vi "NIMS_NS_iir_lpnorm.vi"(5 "Function name":string, 6 "Line number":i32, 7 "Number of outputs requested":i32, 8 "error in (no error)":errorcluster, 11 "[A]":variant[](array[variant])) -> (0 "error out":errorcluster, 3 "[funct(A)]":variant[](array[variant]))   [LabVIEW 2017]
uses:
  <vilib>/imath/engines/lvmath/Functions/Error Handling/error.ctl
  <instcachedir>/0/NIMS_RunTimeType_From StrictType (excl LVString)_1019F277F0A747EDBCA0F6C52CA54500.lvgen/NIMS_RunTimeType_From StrictType (excl LVString)_1019F277F0A747EDBCA0F6C52CA54500_000.vi
  <instcachedir>/0/NIMS_Get Scalar_w Error_1987D997E87247DDAC16EA23A5E9E4FC.lvgen/NIMS_Get Scalar_w Error_1987D997E87247DDAC16EA23A5E9E4FC_000.vi
  <instcachedir>/0/NIMS_Complex To Real_BE01396FDE034E8E94CEBBA1E368668D.lvgen/NIMS_Complex To Real_BE01396FDE034E8E94CEBBA1E368668D_000.vi
  <instcachedir>/0/NIMS_Get Any Vector_w Error - Matrix_9FDB8FBE264C42EDBC8FF9BA66C3EF33.lvgen/NIMS_Get Any Vector_w Error - Matrix_9FDB8FBE264C42EDBC8FF9BA66C3EF33_001.vi
  <instcachedir>/0/NIMS_RunTimeType_To Numeric_1CBDAFC4EFAD4045A1DE52278D16738D.lvgen/NIMS_RunTimeType_To Numeric_1CBDAFC4EFAD4045A1DE52278D16738D_000.vi
  <vilib>/addons/Digital Filter Design/NI_DigFilter_MathScript.lvlib
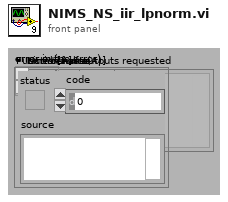
[diagram p1: front panel]
types:
  T1 = typedef "error.ctl" = enum16{"No Error", "Problem", "Input type must not be void", "Incorrect number of parameters", "Function not defined for non-numeric types", "An output variable of the user-defined function is undefined", "Function only defined for character arrays", "Function not defined for boolean, character, or single precision", "Function not defined for complex types", "Not a valid operation", "Inputs must be scalar", "Input matrices are not the same size", "Function only available on RT", "Input matrices must be nonnegative integers of the same type", "Arguments must be non-negative integers less than bitmax", "Number to complement must be less than 2^N", "Bit to get is outside range", "Bit to set is outside range", "Input must be real type ", "At least one parameter must be scalar", "Unable to display plug-in data on RT", "Function not defined for higher dimensional matrices", "Invalid attributes", "Wrong Type of Input Arguments", "Wrong Argument Option", "Invalid file identifier", "Indices must be real positive integers", "The variable is not a matrix data type.", "Number of elements must be the same for indices and values", "You cannot replace elements of a matrix with non-matrix data types.", "Cannot resize a 2D matrix with a linear index", "Unknown variable or symbol", "Indices out of range", "Empty matrix deletion can not be used with two indices", "Number of rows and columns must be the same for indices and values.", "Complex cannot be converted to Boolean", "Char cannot be converted to Boolean", "int64 cannot be converted to Boolean", "uint64 cannot be converted to Boolean", "You cannot convert a Boolean to a character.", "Incompatible input size in 3D surface function", "All rows must have the same number of columns", "Incompatible types", "Invalid matrix dimensions", "Dimension must be 1 or 2", "Base must be an integer between 2 and 36", "Invalid input", "Square matrix required", "Function 'timerstart' must be called before 'timerstop'", "Arguments must be positive real", "Step must not be zero", "Wrong number of input arguments", "Wrong number of output arguments", "Too many index arguments", "Input scalar must be >= 0", "Input scalar must be positive", "Input scalar must not be 0", "Input scalar must be in range [0,1]", "Can't use conditionally defined variable that's undefined", "Input must be a vector", "RT Exec Trace Toolkit not licensed", "Empty vector error", "All elements must be in domain [-1,1]", "All real elements of input vector must be >= 0", "All elements of input vector must be positive", "Values of input vectors are not compatible", "DAQmx not installed", "Input vector must be an increasing vector", "Dereferenced field does not exist within the struct", "A vector or matrix of structures must be indexed before it can be dereferenced", "Lenths of two input vectors are not compatible", "Invalid fieldname", "Empty matrix error", "Cannot use '.' on a type other than Struct", "Unused074", "Data type of the struct's field name is invalid", "Using . to dereference data that is not a struct", "Input struct contains invalid type ", "Size of input matrix is incompatible with input size", "Invalid format specifier", "Could not find field within struct", "Bad permutation array", "Mismatched fieldnames", "ode: User Function could not be opened", "ode: User Function signature does not meet ode requirements", "Unused085", "RunTime: MathScript could not be compiled", "Unknown function", "Only scalars and strings supported", "ode: User Function signature has incorrect number of inputs", "ode:User Function signature has incorrect number of outputs", "Range is too large", "End used without variable", "Function not available (RTE)", "Custom user error", "Arguments must be integers less than bitmax", "Shared library not found", "Header file not found", "Shared library already loaded", "Shared library not loaded", "Shared library function not found", "Shared library string return problem", "Problem calling shared library function", "Problem loading shared library from OS", "Problem parsing shared library header file", "Shared library incompatible types", "Shared library unsupported return type", "Shared library function not exported", "Shared library unsupported input type", "Problem unloading shared library from OS", "Function only available from UI", "Function specified in argument is missing", "An internal error has occurred", "Invalid object", "Invalid property", "Read-only property", "A break command has occurred", "A continue command has occurred", "A return command has occurred", "ode: times parameter invalid", "Function specified in argument has incorrect signature", "Function not found in file", "Reserved keyword cannot be defined as variable", "Reserved keyword cannot be defined as a function or script", "Arguments must be string literals", "Function not supported on this platform", "All columns must have the same number of rows", "Function ignored in RTE warning", "Cannot use : as a parameter that is not a variable", "Output can't be coerced to requested type", "Function not supported on current target", "Variable dependent on an unwired function input", "Unused132", "Unused133", "Unused134", "Unused135", "Unused136", "Unused137", "Unused138", "Unused139", "Global/Persistent must only take constants as arguments.", "Varargin must be last input in the function definition.", "Varargout must be last output in the function definition.", "Invalid output type. Cannot output a cell array of any type other than string.", "Invalid output type. Type is a dynamic struct.", "Invalid output type. Type is a struct that has a field whose type is not known until run-time", "Invalid output type. Type is a struct that has a field which is a plot object.", "MathScript parser DLL missing", "MathScript requires LabVIEW Full", "MathScript license is invalid or missing", "Varargout not supported except in assignments."}
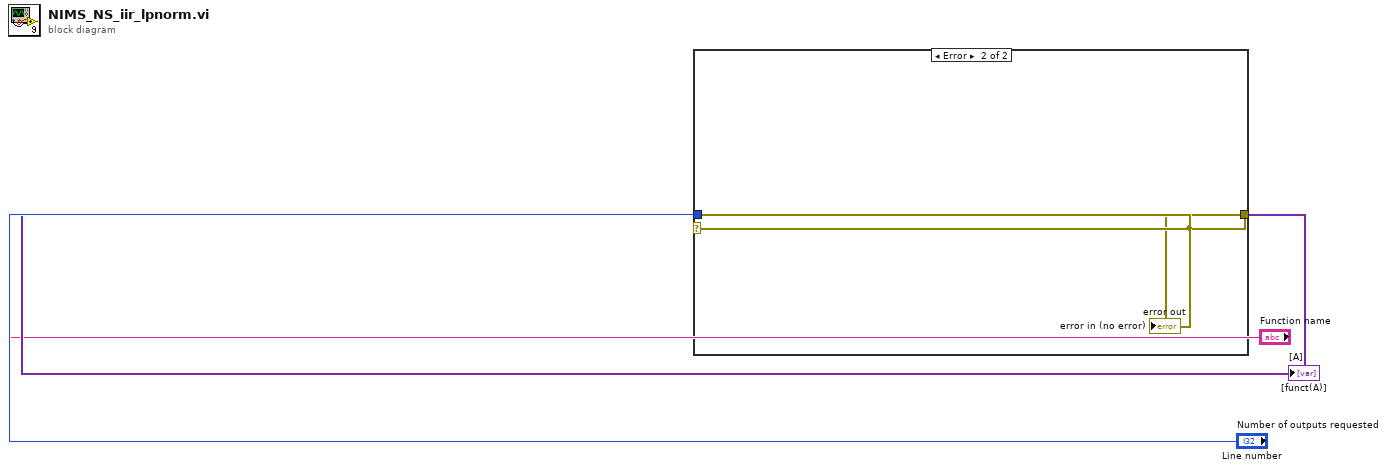
[diagram p0: block diagram]
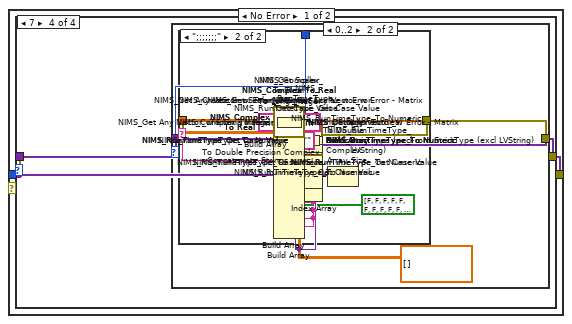
[diagram p2: hidden frame]
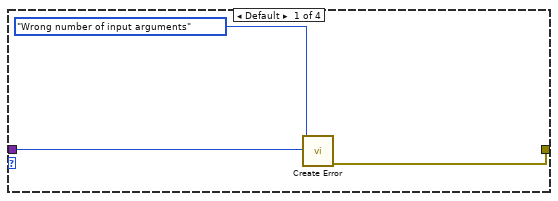
[diagram p3: hidden frame]
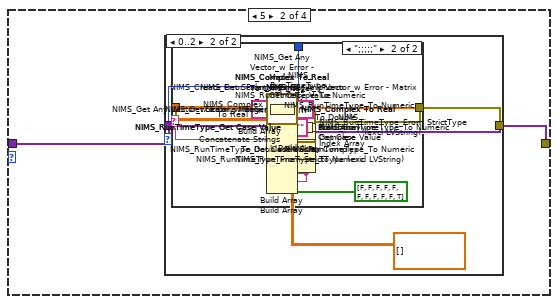
[diagram p4: hidden frame]
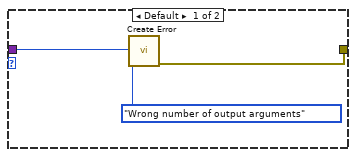
[diagram p5: hidden frame]
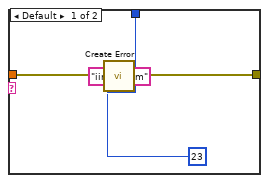
[diagram p6: hidden frame]
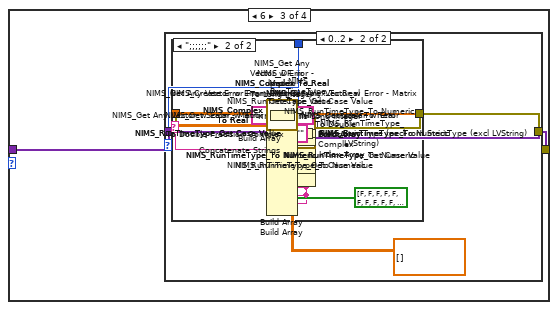
[diagram p7: hidden frame]
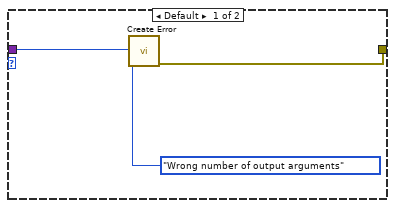
[diagram p8: hidden frame]
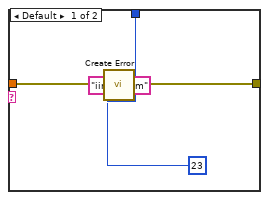
[diagram p9: hidden frame]
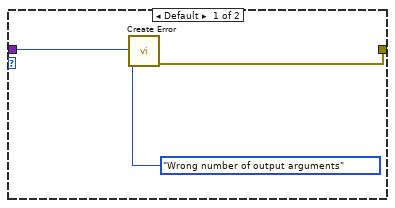
[diagram p10: hidden frame]
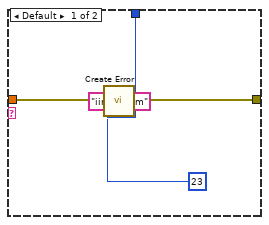
[diagram p11: hidden frame]
diagram:
  n1 = case shown="Error" "error in (no error)" {
    selector: "error in (no error)" -> [_ w322]
    tunnel: [w15 _] -> w4
    tunnel: [w14 w322] -> w3
    tunnel: "error in (no error)" -> [w13 _]
    tunnel: "Number of outputs requested" -> [w12 _]
    tunnel: "[A]" -> [w11 _]
    tunnel: "Function name" -> [w10 _]
    tunnel: "Line number" -> [w9 _]
    frame No Error {
      n2 = Array Size(array=w11) -> (size(s)=w8:i32)
      n3 = case shown="7" w8 {
        tunnel: [_ w27 w118 w218] -> w15
        tunnel: w10 -> [w19 w24 w115 w215]
        tunnel: w9 -> [w20 w25 w116 w216]
        tunnel: w13 -> [w17 w23 w114 w214]
        tunnel: [w16 w22 w113 w213] -> w14
        tunnel: w12 -> [_ w21 w112 w212]
        tunnel: w11 -> [_ w26 w117 w217]
        frame Default {
          n4 = call <vilib>:"Create Error.vi"("Function name"=w19, "error in (no error)"=w17, "Error Enum"=error."Wrong number of input arguments", "Line number"=w20) -> ("error out"=w16:errorcluster)  [unwired: 6 in, 1 out]
        }
        frame 5 {
          n5 = case shown="0..2" w21 {
            tunnel: [_ w33] -> w27
            tunnel: w24 -> [w31 _]
            tunnel: w25 -> [w32 w67]
            tunnel: w23 -> [w29 w65]
            tunnel: [w28 w44] -> w22
            tunnel: w26 -> [_ w68]
            frame Default {
              n6 = call <vilib>:"Create Error.vi"("Function name"=w31, "error in (no error)"=w29, "Error Enum"=error."Wrong number of output arguments", "Line number"=w32) -> ("error out"=w28:errorcluster)  [unwired: 6 in, 1 out]
            }
            frame 0..2 {
              n7 = Index Array(array=w68) -> (element #1=w64:variant, element #2=w60:variant, element #3=w56:variant, element #4=w52:variant, element #5=w48:variant)  [unwired: 5 in]
              n8 = call <vilib>:"NIMS_RunTimeType_Get Case Value.vi"("Data In"=w48) -> ("Case Value"=w45:string)  [unwired: 9 in, 1 out]
              n9 = call-generic <vilib>:"NIMS_RunTimeType_To Numeric.vi"("DataType"=cdb[][] [], "Variant"=w48) -> ("data"=w46:cdb[][])  [unwired: 1 in]
              n10 = call <vilib>:"NIMS_RunTimeType_Get Case Value.vi"("Data In"=w52) -> ("Case Value"=w49:string)  [unwired: 9 in, 1 out]
              n11 = call-generic <vilib>:"NIMS_RunTimeType_To Numeric.vi"("DataType"=cdb[][] [], "Variant"=w52) -> ("data"=w50:cdb[][])  [unwired: 1 in]
              n12 = call <vilib>:"NIMS_RunTimeType_Get Case Value.vi"("Data In"=w56) -> ("Case Value"=w53:string)  [unwired: 9 in, 1 out]
              n13 = call-generic <vilib>:"NIMS_RunTimeType_To Numeric.vi"("DataType"=cdb[][] [], "Variant"=w56) -> ("data"=w54:cdb[][])  [unwired: 1 in]
              n14 = call <vilib>:"NIMS_RunTimeType_Get Case Value.vi"("Data In"=w60) -> ("Case Value"=w57:string)  [unwired: 9 in, 1 out]
              n15 = call-generic <vilib>:"NIMS_RunTimeType_To Numeric.vi"("DataType"=cdb[][] [], "Variant"=w60) -> ("data"=w58:cdb[][])  [unwired: 1 in]
              n16 = call <vilib>:"NIMS_RunTimeType_Get Case Value.vi"("Data In"=w64) -> ("Case Value"=w61:string)  [unwired: 9 in, 1 out]
              n17 = call-generic <vilib>:"NIMS_RunTimeType_To Numeric.vi"("DataType"=cdb[][] [], "Variant"=w64) -> ("data"=w62:cdb[][])  [unwired: 1 in]
              n18 = Concatenate Strings(w61, w57, w53, w49, w45) -> (w66:string)
              n19 = case shown="\";;;;;\"" w66 {
                tunnel: w65 -> [w70 w80]
                tunnel: [_ w75] -> w43
                tunnel: [_ w74] -> w39
                tunnel: [w69 w76] -> w44
                tunnel: w62 -> [_ w110]
                tunnel: w58 -> [_ w106]
                tunnel: w54 -> [_ w102]
                tunnel: w50 -> [_ w99]
                tunnel: w46 -> [_ w96]
                tunnel: w67 -> [w73 w83]
                frame Default {
                  n20 = call <vilib>:"Create Error.vi"("Function name"="iir_lpnorm", "error in (no error)"=w70, "Error Enum"=23, "Line number"=w73) -> ("error out"=w69:errorcluster)  [unwired: 6 in, 1 out]
                }
                frame ";;;;;" {
                  w78 = "iir_lpnorm"
                  n21 = call-generic <vilib>:"NIMS_Complex To Real.vi"("A"=w96) -> ("Error Enum"=w86:T1, "Real(A)"=w95:dbl[][])  [unwired: 8 in, 1 out]
                  n22 = call-generic <vilib>:"NIMS_Get Any Vector_w Error - Matrix.vi"("A"=w95) -> ("Error Enum"=w85:T1, "Vector"=w97:dbl[])  [unwired: 8 in, 1 out]
                  n23 = call-generic <vilib>:"NIMS_Complex To Real.vi"("A"=w99) -> ("Error Enum"=w88:T1, "Real(A)"=w98:dbl[][])  [unwired: 8 in, 1 out]
                  n24 = call-generic <vilib>:"NIMS_Get Any Vector_w Error - Matrix.vi"("A"=w98) -> ("Error Enum"=w87:T1, "Vector"=w100:dbl[])  [unwired: 8 in, 1 out]
                  n25 = call-generic <vilib>:"NIMS_Complex To Real.vi"("A"=w102) -> ("Error Enum"=w90:T1, "Real(A)"=w101:dbl[][])  [unwired: 8 in, 1 out]
                  n26 = call-generic <vilib>:"NIMS_Get Any Vector_w Error - Matrix.vi"("A"=w101) -> ("Error Enum"=w89:T1, "Vector"=w103:dbl[])  [unwired: 8 in, 1 out]
                  n27 = call-generic <vilib>:"NIMS_Complex To Real.vi"("A"=w106) -> ("Error Enum"=w92:T1, "Real(A)"=w105:dbl[][])  [unwired: 8 in, 1 out]
                  n28 = To Long Integer(number=w105) -> (32bit integer=w104:i32[][])
                  n29 = call-generic <vilib>:"NIMS_Get Scalar_w Error.vi"("A"=w104) -> ("Error Enum"=w91:T1, "Scalar"=w107:i32)  [unwired: 8 in, 1 out]
                  n30 = call-generic <vilib>:"NIMS_Complex To Real.vi"("A"=w110) -> ("Error Enum"=w94:T1, "Real(A)"=w109:dbl[][])  [unwired: 8 in, 1 out]
                  n31 = To Long Integer(number=w109) -> (32bit integer=w108:i32[][])
                  n32 = call-generic <vilib>:"NIMS_Get Scalar_w Error.vi"("A"=w108) -> ("Error Enum"=w93:T1, "Scalar"=w111:i32)  [unwired: 8 in, 1 out]
                  n33 = call <vilib>:"NIMS_DF_iir_lpnorm.vi"("mag"=w97, "e"=w100, "f"=w103, "d"=w107, "n"=w111) -> ("error"=w84:i32, "a"=w74:dbl[], "b"=w75:dbl[])  [unwired: 4 in]
                  n34 = Build Array(w78, w78, w78, w78, w78, w78, w78, w78, w78, w78, "iir_lpnorm") -> (w81:string[])
                  n35 = Build Array(w94, w93, w92, w91, w90, w89, w88, w87, w86, w85, w84) -> (w82:i32[])
                  n36 = call <vilib>:"NIMS_Create Error From Enums.vi"("Error Code"=bool[] [FALSE, FALSE, FALSE, FALSE, FALSE, FALSE, FALSE, FALSE, FALSE, FALSE, TRUE], "error in (no error)"=w80, "Line no"=w83, "Error Enums"=w82, "Function names"=w81) -> ("error out"=w76:errorcluster)  [unwired: 6 in]
                }
              }
              n37 = Build Array(w39) -> (w38:dbl[][])
              n38 = To Double Precision Complex(1:w38) -> (0:w37:cdb[][])
              n39 = call-generic <vilib>:"NIMS_RunTimeType_From StrictType (excl LVString).vi"("Plug-In Name"="", "Data In"=w37) -> ("Data Out"=w34:variant)  [unwired: 2 in]
              n40 = Build Array(w43) -> (w42:dbl[][])
              n41 = To Double Precision Complex(1:w42) -> (0:w41:cdb[][])
              n42 = call-generic <vilib>:"NIMS_RunTimeType_From StrictType (excl LVString).vi"("Plug-In Name"="", "Data In"=w41) -> ("Data Out"=w35:variant)  [unwired: 2 in]
              n43 = Build Array(w35, w34) -> (w33:variant[])
            }
          }
        }
        frame 6 {
          n44 = case shown="0..2" w112 {
            tunnel: [_ w124] -> w118
            tunnel: w115 -> [w122 _]
            tunnel: w116 -> [w123 w162]
            tunnel: w114 -> [w120 w160]
            tunnel: [w119 w135] -> w113
            tunnel: w117 -> [_ w163]
            frame Default {
              n45 = call <vilib>:"Create Error.vi"("Function name"=w122, "error in (no error)"=w120, "Error Enum"=error."Wrong number of output arguments", "Line number"=w123) -> ("error out"=w119:errorcluster)  [unwired: 6 in, 1 out]
            }
            frame 0..2 {
              n46 = Index Array(array=w163) -> (element #1=w159:variant, element #2=w155:variant, element #3=w151:variant, element #4=w147:variant, element #5=w143:variant, element #6=w139:variant)  [unwired: 6 in]
              n47 = call <vilib>:"NIMS_RunTimeType_Get Case Value.vi"("Data In"=w139) -> ("Case Value"=w136:string)  [unwired: 9 in, 1 out]
              n48 = call-generic <vilib>:"NIMS_RunTimeType_To Numeric.vi"("DataType"=cdb[][] [], "Variant"=w139) -> ("data"=w137:cdb[][])  [unwired: 1 in]
              n49 = call <vilib>:"NIMS_RunTimeType_Get Case Value.vi"("Data In"=w143) -> ("Case Value"=w140:string)  [unwired: 9 in, 1 out]
              n50 = call-generic <vilib>:"NIMS_RunTimeType_To Numeric.vi"("DataType"=cdb[][] [], "Variant"=w143) -> ("data"=w141:cdb[][])  [unwired: 1 in]
              n51 = call <vilib>:"NIMS_RunTimeType_Get Case Value.vi"("Data In"=w147) -> ("Case Value"=w144:string)  [unwired: 9 in, 1 out]
              n52 = call-generic <vilib>:"NIMS_RunTimeType_To Numeric.vi"("DataType"=cdb[][] [], "Variant"=w147) -> ("data"=w145:cdb[][])  [unwired: 1 in]
              n53 = call <vilib>:"NIMS_RunTimeType_Get Case Value.vi"("Data In"=w151) -> ("Case Value"=w148:string)  [unwired: 9 in, 1 out]
              n54 = call-generic <vilib>:"NIMS_RunTimeType_To Numeric.vi"("DataType"=cdb[][] [], "Variant"=w151) -> ("data"=w149:cdb[][])  [unwired: 1 in]
              n55 = call <vilib>:"NIMS_RunTimeType_Get Case Value.vi"("Data In"=w155) -> ("Case Value"=w152:string)  [unwired: 9 in, 1 out]
              n56 = call-generic <vilib>:"NIMS_RunTimeType_To Numeric.vi"("DataType"=cdb[][] [], "Variant"=w155) -> ("data"=w153:cdb[][])  [unwired: 1 in]
              n57 = call <vilib>:"NIMS_RunTimeType_Get Case Value.vi"("Data In"=w159) -> ("Case Value"=w156:string)  [unwired: 9 in, 1 out]
              n58 = call-generic <vilib>:"NIMS_RunTimeType_To Numeric.vi"("DataType"=cdb[][] [], "Variant"=w159) -> ("data"=w157:cdb[][])  [unwired: 1 in]
              n59 = Concatenate Strings(w156, w152, w148, w144, w140, w136) -> (w161:string)
              n60 = case shown="\";;;;;;\"" w161 {
                tunnel: w160 -> [w165 w175]
                tunnel: [_ w170] -> w134
                tunnel: [_ w169] -> w130
                tunnel: [w164 w171] -> w135
                tunnel: w157 -> [_ w210]
                tunnel: w153 -> [_ w206]
                tunnel: w149 -> [_ w202]
                tunnel: w145 -> [_ w199]
                tunnel: w141 -> [_ w196]
                tunnel: w137 -> [_ w193]
                tunnel: w162 -> [w168 w178]
                frame Default {
                  n61 = call <vilib>:"Create Error.vi"("Function name"="iir_lpnorm", "error in (no error)"=w165, "Error Enum"=23, "Line number"=w168) -> ("error out"=w164:errorcluster)  [unwired: 6 in, 1 out]
                }
                frame ";;;;;;" {
                  w173 = "iir_lpnorm"
                  n62 = call-generic <vilib>:"NIMS_Complex To Real.vi"("A"=w193) -> ("Error Enum"=w181:T1, "Real(A)"=w192:dbl[][])  [unwired: 8 in, 1 out]
                  n63 = call-generic <vilib>:"NIMS_Get Any Vector_w Error - Matrix.vi"("A"=w192) -> ("Error Enum"=w180:T1, "Vector"=w194:dbl[])  [unwired: 8 in, 1 out]
                  n64 = call-generic <vilib>:"NIMS_Complex To Real.vi"("A"=w196) -> ("Error Enum"=w183:T1, "Real(A)"=w195:dbl[][])  [unwired: 8 in, 1 out]
                  n65 = call-generic <vilib>:"NIMS_Get Any Vector_w Error - Matrix.vi"("A"=w195) -> ("Error Enum"=w182:T1, "Vector"=w197:dbl[])  [unwired: 8 in, 1 out]
                  n66 = call-generic <vilib>:"NIMS_Complex To Real.vi"("A"=w199) -> ("Error Enum"=w185:T1, "Real(A)"=w198:dbl[][])  [unwired: 8 in, 1 out]
                  n67 = call-generic <vilib>:"NIMS_Get Any Vector_w Error - Matrix.vi"("A"=w198) -> ("Error Enum"=w184:T1, "Vector"=w200:dbl[])  [unwired: 8 in, 1 out]
                  n68 = call-generic <vilib>:"NIMS_Complex To Real.vi"("A"=w202) -> ("Error Enum"=w187:T1, "Real(A)"=w201:dbl[][])  [unwired: 8 in, 1 out]
                  n69 = call-generic <vilib>:"NIMS_Get Any Vector_w Error - Matrix.vi"("A"=w201) -> ("Error Enum"=w186:T1, "Vector"=w203:dbl[])  [unwired: 8 in, 1 out]
                  n70 = call-generic <vilib>:"NIMS_Complex To Real.vi"("A"=w206) -> ("Error Enum"=w189:T1, "Real(A)"=w205:dbl[][])  [unwired: 8 in, 1 out]
                  n71 = To Long Integer(number=w205) -> (32bit integer=w204:i32[][])
                  n72 = call-generic <vilib>:"NIMS_Get Scalar_w Error.vi"("A"=w204) -> ("Error Enum"=w188:T1, "Scalar"=w207:i32)  [unwired: 8 in, 1 out]
                  n73 = call-generic <vilib>:"NIMS_Complex To Real.vi"("A"=w210) -> ("Error Enum"=w191:T1, "Real(A)"=w209:dbl[][])  [unwired: 8 in, 1 out]
                  n74 = To Long Integer(number=w209) -> (32bit integer=w208:i32[][])
                  n75 = call-generic <vilib>:"NIMS_Get Scalar_w Error.vi"("A"=w208) -> ("Error Enum"=w190:T1, "Scalar"=w211:i32)  [unwired: 8 in, 1 out]
                  n76 = call <vilib>:"NIMS_DF_iir_lpnorm.vi"("w"=w194, "mag"=w197, "e"=w200, "f"=w203, "d"=w207, "n"=w211) -> ("error"=w179:i32, "a"=w169:dbl[], "b"=w170:dbl[])  [unwired: 3 in]
                  n77 = Build Array(w173, w173, w173, w173, w173, w173, w173, w173, w173, w173, w173, w173, "iir_lpnorm") -> (w176:string[])
                  n78 = Build Array(w191, w190, w189, w188, w187, w186, w185, w184, w183, w182, w181, w180, w179) -> (w177:i32[])
                  n79 = call <vilib>:"NIMS_Create Error From Enums.vi"("Error Code"=bool[] [FALSE, FALSE, FALSE, FALSE, FALSE, FALSE, FALSE, FALSE, FALSE, FALSE, FALSE, FALSE, TRUE], "error in (no error)"=w175, "Line no"=w178, "Error Enums"=w177, "Function names"=w176) -> ("error out"=w171:errorcluster)  [unwired: 6 in]
                }
              }
              n80 = Build Array(w130) -> (w129:dbl[][])
              n81 = To Double Precision Complex(1:w129) -> (0:w128:cdb[][])
              n82 = call-generic <vilib>:"NIMS_RunTimeType_From StrictType (excl LVString).vi"("Plug-In Name"="", "Data In"=w128) -> ("Data Out"=w125:variant)  [unwired: 2 in]
              n83 = Build Array(w134) -> (w133:dbl[][])
              n84 = To Double Precision Complex(1:w133) -> (0:w132:cdb[][])
              n85 = call-generic <vilib>:"NIMS_RunTimeType_From StrictType (excl LVString).vi"("Plug-In Name"="", "Data In"=w132) -> ("Data Out"=w126:variant)  [unwired: 2 in]
              n86 = Build Array(w126, w125) -> (w124:variant[])
            }
          }
        }
        frame 7 {
          n87 = case shown="0..2" w212 {
            tunnel: [_ w224] -> w218
            tunnel: w215 -> [w222 _]
            tunnel: w216 -> [w223 w266]
            tunnel: w214 -> [w220 w264]
            tunnel: [w219 w235] -> w213
            tunnel: w217 -> [_ w267]
            frame Default {
              n88 = call <vilib>:"Create Error.vi"("Function name"=w222, "error in (no error)"=w220, "Error Enum"=error."Wrong number of output arguments", "Line number"=w223) -> ("error out"=w219:errorcluster)  [unwired: 6 in, 1 out]
            }
            frame 0..2 {
              n89 = Index Array(array=w267) -> (element #1=w263:variant, element #2=w259:variant, element #3=w255:variant, element #4=w251:variant, element #5=w247:variant, element #6=w243:variant, element #7=w239:variant)  [unwired: 7 in]
              n90 = call <vilib>:"NIMS_RunTimeType_Get Case Value.vi"("Data In"=w239) -> ("Case Value"=w236:string)  [unwired: 9 in, 1 out]
              n91 = call-generic <vilib>:"NIMS_RunTimeType_To Numeric.vi"("DataType"=cdb[][] [], "Variant"=w239) -> ("data"=w237:cdb[][])  [unwired: 1 in]
              n92 = call <vilib>:"NIMS_RunTimeType_Get Case Value.vi"("Data In"=w243) -> ("Case Value"=w240:string)  [unwired: 9 in, 1 out]
              n93 = call-generic <vilib>:"NIMS_RunTimeType_To Numeric.vi"("DataType"=cdb[][] [], "Variant"=w243) -> ("data"=w241:cdb[][])  [unwired: 1 in]
              n94 = call <vilib>:"NIMS_RunTimeType_Get Case Value.vi"("Data In"=w247) -> ("Case Value"=w244:string)  [unwired: 9 in, 1 out]
              n95 = call-generic <vilib>:"NIMS_RunTimeType_To Numeric.vi"("DataType"=cdb[][] [], "Variant"=w247) -> ("data"=w245:cdb[][])  [unwired: 1 in]
              n96 = call <vilib>:"NIMS_RunTimeType_Get Case Value.vi"("Data In"=w251) -> ("Case Value"=w248:string)  [unwired: 9 in, 1 out]
              n97 = call-generic <vilib>:"NIMS_RunTimeType_To Numeric.vi"("DataType"=cdb[][] [], "Variant"=w251) -> ("data"=w249:cdb[][])  [unwired: 1 in]
              n98 = call <vilib>:"NIMS_RunTimeType_Get Case Value.vi"("Data In"=w255) -> ("Case Value"=w252:string)  [unwired: 9 in, 1 out]
              n99 = call-generic <vilib>:"NIMS_RunTimeType_To Numeric.vi"("DataType"=cdb[][] [], "Variant"=w255) -> ("data"=w253:cdb[][])  [unwired: 1 in]
              n100 = call <vilib>:"NIMS_RunTimeType_Get Case Value.vi"("Data In"=w259) -> ("Case Value"=w256:string)  [unwired: 9 in, 1 out]
              n101 = call-generic <vilib>:"NIMS_RunTimeType_To Numeric.vi"("DataType"=cdb[][] [], "Variant"=w259) -> ("data"=w257:cdb[][])  [unwired: 1 in]
              n102 = call <vilib>:"NIMS_RunTimeType_Get Case Value.vi"("Data In"=w263) -> ("Case Value"=w260:string)  [unwired: 9 in, 1 out]
              n103 = call-generic <vilib>:"NIMS_RunTimeType_To Numeric.vi"("DataType"=cdb[][] [], "Variant"=w263) -> ("data"=w261:cdb[][])  [unwired: 1 in]
              n104 = Concatenate Strings(w260, w256, w252, w248, w244, w240, w236) -> (w265:string)
              n105 = case shown="\";;;;;;;\"" w265 {
                tunnel: w264 -> [w269 w279]
                tunnel: [_ w274] -> w234
                tunnel: [_ w273] -> w230
                tunnel: [w268 w275] -> w235
                tunnel: w261 -> [_ w320]
                tunnel: w257 -> [_ w316]
                tunnel: w253 -> [_ w312]
                tunnel: w249 -> [_ w309]
                tunnel: w245 -> [_ w306]
                tunnel: w241 -> [_ w303]
                tunnel: w237 -> [_ w300]
                tunnel: w266 -> [w272 w282]
                frame Default {
                  n106 = call <vilib>:"Create Error.vi"("Function name"="iir_lpnorm", "error in (no error)"=w269, "Error Enum"=23, "Line number"=w272) -> ("error out"=w268:errorcluster)  [unwired: 6 in, 1 out]
                }
                frame ";;;;;;;" {
                  w277 = "iir_lpnorm"
                  n107 = call-generic <vilib>:"NIMS_Complex To Real.vi"("A"=w300) -> ("Error Enum"=w285:T1, "Real(A)"=w299:dbl[][])  [unwired: 8 in, 1 out]
                  n108 = To Long Integer(number=w299) -> (32bit integer=w298:i32[][])
                  n109 = call-generic <vilib>:"NIMS_Get Scalar_w Error.vi"("A"=w298) -> ("Error Enum"=w284:T1, "Scalar"=w301:i32)  [unwired: 8 in, 1 out]
                  n110 = call-generic <vilib>:"NIMS_Complex To Real.vi"("A"=w303) -> ("Error Enum"=w287:T1, "Real(A)"=w302:dbl[][])  [unwired: 8 in, 1 out]
                  n111 = call-generic <vilib>:"NIMS_Get Any Vector_w Error - Matrix.vi"("A"=w302) -> ("Error Enum"=w286:T1, "Vector"=w304:dbl[])  [unwired: 8 in, 1 out]
                  n112 = call-generic <vilib>:"NIMS_Complex To Real.vi"("A"=w306) -> ("Error Enum"=w289:T1, "Real(A)"=w305:dbl[][])  [unwired: 8 in, 1 out]
                  n113 = call-generic <vilib>:"NIMS_Get Any Vector_w Error - Matrix.vi"("A"=w305) -> ("Error Enum"=w288:T1, "Vector"=w307:dbl[])  [unwired: 8 in, 1 out]
                  n114 = call-generic <vilib>:"NIMS_Complex To Real.vi"("A"=w309) -> ("Error Enum"=w291:T1, "Real(A)"=w308:dbl[][])  [unwired: 8 in, 1 out]
                  n115 = call-generic <vilib>:"NIMS_Get Any Vector_w Error - Matrix.vi"("A"=w308) -> ("Error Enum"=w290:T1, "Vector"=w310:dbl[])  [unwired: 8 in, 1 out]
                  n116 = call-generic <vilib>:"NIMS_Complex To Real.vi"("A"=w312) -> ("Error Enum"=w293:T1, "Real(A)"=w311:dbl[][])  [unwired: 8 in, 1 out]
                  n117 = call-generic <vilib>:"NIMS_Get Any Vector_w Error - Matrix.vi"("A"=w311) -> ("Error Enum"=w292:T1, "Vector"=w313:dbl[])  [unwired: 8 in, 1 out]
                  n118 = call-generic <vilib>:"NIMS_Complex To Real.vi"("A"=w316) -> ("Error Enum"=w295:T1, "Real(A)"=w315:dbl[][])  [unwired: 8 in, 1 out]
                  n119 = To Long Integer(number=w315) -> (32bit integer=w314:i32[][])
                  n120 = call-generic <vilib>:"NIMS_Get Scalar_w Error.vi"("A"=w314) -> ("Error Enum"=w294:T1, "Scalar"=w317:i32)  [unwired: 8 in, 1 out]
                  n121 = call-generic <vilib>:"NIMS_Complex To Real.vi"("A"=w320) -> ("Error Enum"=w297:T1, "Real(A)"=w319:dbl[][])  [unwired: 8 in, 1 out]
                  n122 = To Long Integer(number=w319) -> (32bit integer=w318:i32[][])
                  n123 = call-generic <vilib>:"NIMS_Get Scalar_w Error.vi"("A"=w318) -> ("Error Enum"=w296:T1, "Scalar"=w321:i32)  [unwired: 8 in, 1 out]
                  n124 = call <vilib>:"NIMS_DF_iir_lpnorm.vi"("p"=w301, "w"=w304, "mag"=w307, "e"=w310, "f"=w313, "d"=w317, "n"=w321) -> ("error"=w283:i32, "a"=w273:dbl[], "b"=w274:dbl[])  [unwired: 2 in]
                  n125 = Build Array(w277, w277, w277, w277, w277, w277, w277, w277, w277, w277, w277, w277, w277, w277, "iir_lpnorm") -> (w280:string[])
                  n126 = Build Array(w297, w296, w295, w294, w293, w292, w291, w290, w289, w288, w287, w286, w285, w284, w283) -> (w281:i32[])
                  n127 = call <vilib>:"NIMS_Create Error From Enums.vi"("Error Code"=bool[] [FALSE, FALSE, FALSE, FALSE, FALSE, FALSE, FALSE, FALSE, FALSE, FALSE, FALSE, FALSE, FALSE, FALSE, TRUE], "error in (no error)"=w279, "Line no"=w282, "Error Enums"=w281, "Function names"=w280) -> ("error out"=w275:errorcluster)  [unwired: 6 in]
                }
              }
              n128 = Build Array(w230) -> (w229:dbl[][])
              n129 = To Double Precision Complex(1:w229) -> (0:w228:cdb[][])
              n130 = call-generic <vilib>:"NIMS_RunTimeType_From StrictType (excl LVString).vi"("Plug-In Name"="", "Data In"=w228) -> ("Data Out"=w225:variant)  [unwired: 2 in]
              n131 = Build Array(w234) -> (w233:dbl[][])
              n132 = To Double Precision Complex(1:w233) -> (0:w232:cdb[][])
              n133 = call-generic <vilib>:"NIMS_RunTimeType_From StrictType (excl LVString).vi"("Plug-In Name"="", "Data In"=w232) -> ("Data Out"=w226:variant)  [unwired: 2 in]
              n134 = Build Array(w226, w225) -> (w224:variant[])
            }
          }
        }
      }
    }
    frame Error {
    }
  }
  "error out" <- w3
  "[funct(A)]" <- w4
